vi "AmpPolNames.vi"(0 "Polarity array":refnum<vi>[](array[refnum]), 1 "Amplitude array":refnum<vi>[](array[refnum])) -> (2 "Array 2":enum16{"Negative", "Positive"}[](array[ring]), 3 "Array 3":dbl[](array[numeric]), 4 "Array 4":string[](array[string]), 5 "Array":string[][](array[string]))   [LabVIEW 2013]
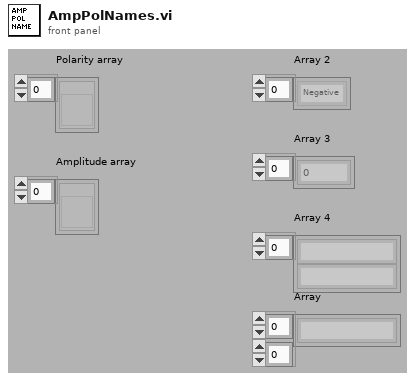
[diagram p1: front panel]
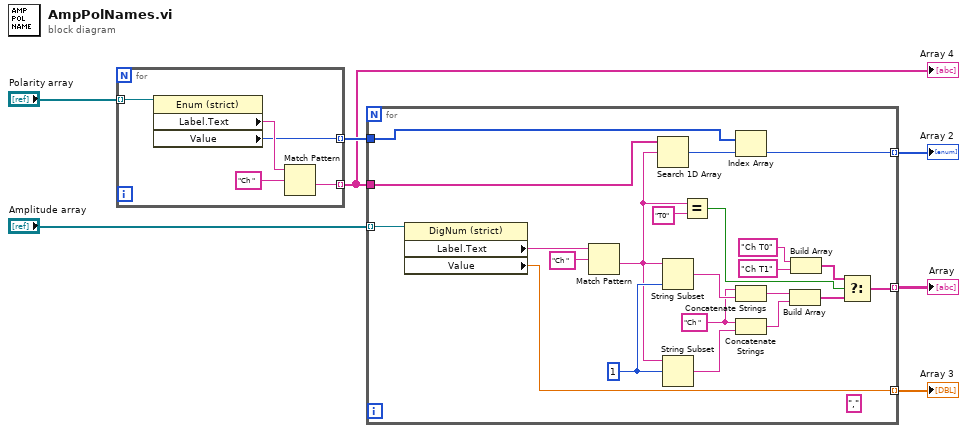
[diagram p0: block diagram]
diagram:
  n1 = for {
    tunnel: "Polarity array" -> [w12] mode=indexing
    tunnel: [w9] -> w2 mode=indexing
    tunnel: [w8] -> w3 mode=indexing
    n2 = property class="Enum (strict)"(reference=w12) -> ("Label.Text"=w10:string, "Value"=w8:enum16{"Negative", "Positive"})  [unwired: 1 in, 2 out]
    n3 = Match Pattern(string=w10, regular expression="Ch ") -> (after substring=w9:string)  [unwired: 1 in, 3 out]
  }
  "Array 4" <- w2
  n4 = for {
    tunnel: "Amplitude array" -> [w34] mode=indexing
    tunnel: [w27] -> w6 mode=indexing
    tunnel: [w18] -> w4 mode=indexing
    tunnel: w2 -> [w17]
    tunnel: w3 -> [w15]
    tunnel: [w13] -> w5 mode=indexing
    w23 = "Ch " ("string")
    (unwired) "," ("string")
    w29 = 1 ("offset (0)")
    n5 = property class="DigNum (strict)"(reference=w34) -> ("Label.Text"=w32:string, "Value"=w18:dbl)  [unwired: 1 in, 2 out]
    n6 = Match Pattern(string=w32, regular expression="Ch ") -> (after substring=w16:string)  [unwired: 1 in, 3 out]
    n7 = Search 1D Array(1D array=w17, element=w16) -> (index of element=w14:i32)  [unwired: 1 in]
    n8 = String Subset(string=w16, length (rest)=w29) -> (substring=w28:string)  [unwired: 1 in]
    n9 = String Subset(string=w16, offset (0)=w29) -> (substring=w22:string)  [unwired: 1 in]
    n10 = Equal?(x=w16, y="T0") -> (x = y?=w31:bool)
    n11 = Index Array(array=w15, index=w14) -> (element=w13:enum16{"Negative", "Positive"})
    n12 = Concatenate Strings(w23, w28) -> (w20:string)
    n13 = Concatenate Strings(w23, w22) -> (w19:string)
    n14 = Build Array(w20, w19) -> (w21:string[])
    n15 = Build Array("Ch T0" ("t"), "Ch T1" ("t")) -> (w24:string[])
    n16 = Select(t=w24, s=w31, f=w21) -> (s? t:f=w27:string[])
  }
  "Array" <- w6
  "Array 2" <- w5
  "Array 3" <- w4
